vi "Get Divisors.vi"(11 "Number":i32) -> (3 "Divisors":i32[](array[numeric]))   [LabVIEW 2013, in "Problem 21.lvlib"]
uses:
  Problem 21.lvlib
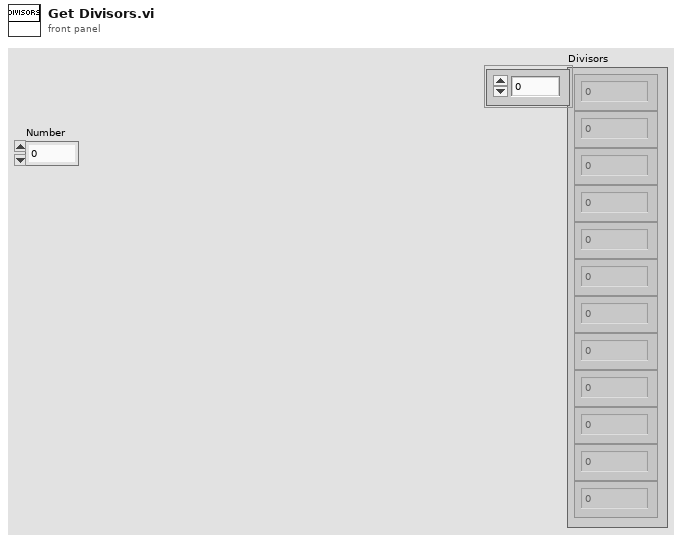
[diagram p1: front panel]
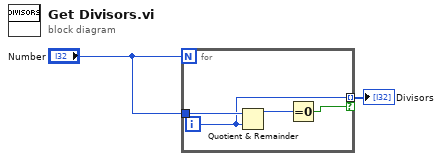
[diagram p0: block diagram]
diagram:
  n1 = for {
    N: "Number" -> [_]
    tunnel: "Number" -> [w6]
    tunnel: [w3] -> w1 mode=indexing if=w4
    i -> [w3]
    n2 = Quotient & Remainder(x=w6, y=w3) -> (x-y*floor(x/y)=w5:i32)  [unwired: 1 out]
    n3 = Equal To 0?(x=w5) -> (x = 0?=w4:bool)
  }
  "Divisors" <- w1
